vi "Write Element of VI refs.vi"(8 "error in (no error)":errorcluster, 9 "vi reference":refnum<vi>, 10 "name":string, 11 "Control-Client in":refnum<class "Control-Client.lvclass">) -> (0 "error out":errorcluster, 3 "Control-Client out":refnum<class "Control-Client.lvclass">)   [LabVIEW 2019, in "Control-Client.lvclass"]
uses:
  Control-Client.lvclass
  Control-Client.lvclass/Control-Client.ctl
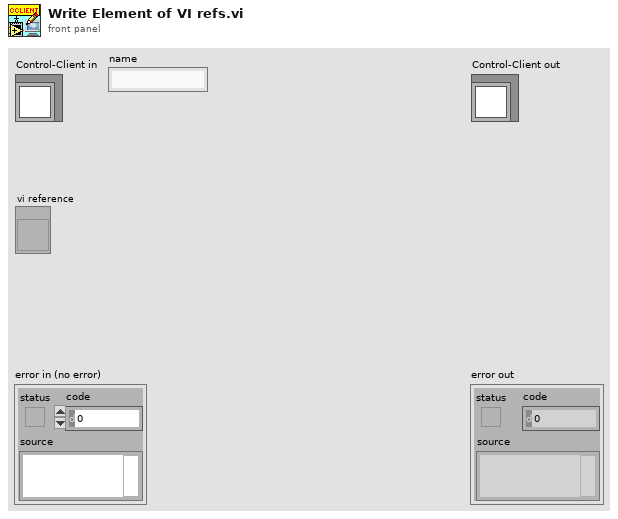
[diagram p1: front panel]
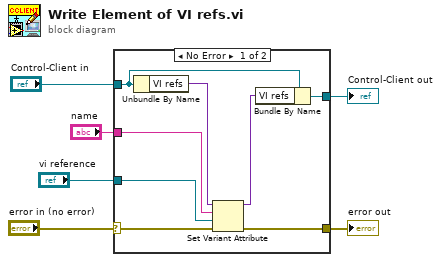
[diagram p0: block diagram]
diagram:
  n1 = case shown="No Error" "error in (no error)" {
    selector: "error in (no error)" -> [w8 w15]
    tunnel: [w7 w15] -> w5
    tunnel: [w14 w16] -> w3
    tunnel: "Control-Client in" -> [w13 w16]
    tunnel: "vi reference" -> [w9 _]
    tunnel: "name" -> [w10 _]
    frame No Error {
      n2 = Unbundle By Name(w13) -> ("VI refs"=w12:variant)
      n3 = Set Variant Attribute(Variant=w12, name=w10, value=w9, error in=w8) -> (Variant out=w11:variant, error out=w7:errorcluster)  [unwired: 1 out]
      n4 = Bundle By Name(cluster=w13, "VI refs"=w11) -> (w14:refnum<class "Control-Client.lvclass">)
    }
    frame Error {
    }
  }
  "error out" <- w5
  "Control-Client out" <- w3
